vi "ConfigUtilities - Configure Packet Header.vi"(8 "error in (no error)":errorcluster, 9 "Header Elements In":bool[](array[boolean]), 11 "Packet Ref in":T1 format="%.0x") -> (0 "error out":errorcluster, 1 "Header Elements Out":bool[](array[boolean]), 3 "Packet Ref out":T1 format="%.0x")   [LabVIEW 2016, in "UDP-Custom-Device System Explorer.lvlib"]
uses:
  UDP-Custom-Device System Explorer.lvlib
  <vilib>/NI Veristand/Custom Device API/Custom Device Item Ref.ctl
  <vilib>/NI VeriStand/Custom Device API/Custom Device API.lvlib
panel:
  in  "TimeStamp":bool
  out "Data Header":string="Data"
  out "Num Bits Header":string="Num Bits"
  out "Data":string
  out "Num Bits":string
  in  "Cancel":bool
  in  "OK":bool
  in  "Packet Sequence":bool
  in  "Packet ID":bool
  in  "Num of Chans":bool
  # "Select Packet Header Information"
  # "Sample Packet Header"
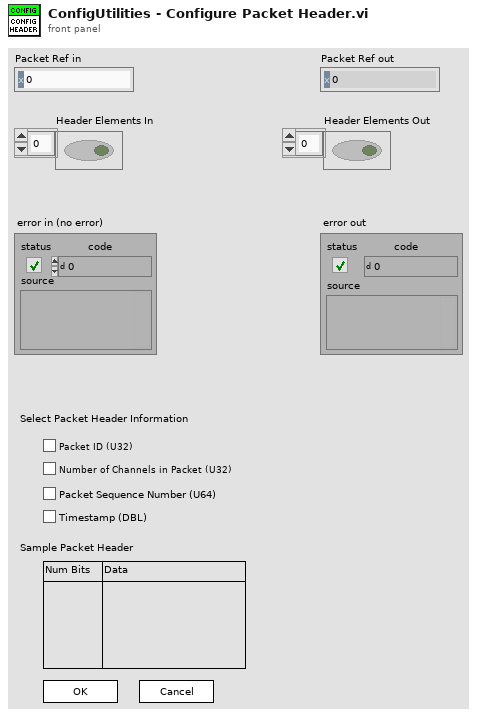
[diagram p1: front panel]
types:
  T1 = typedef "Custom Device API.lvlib/Custom Device Item Ref.ctl" = u64
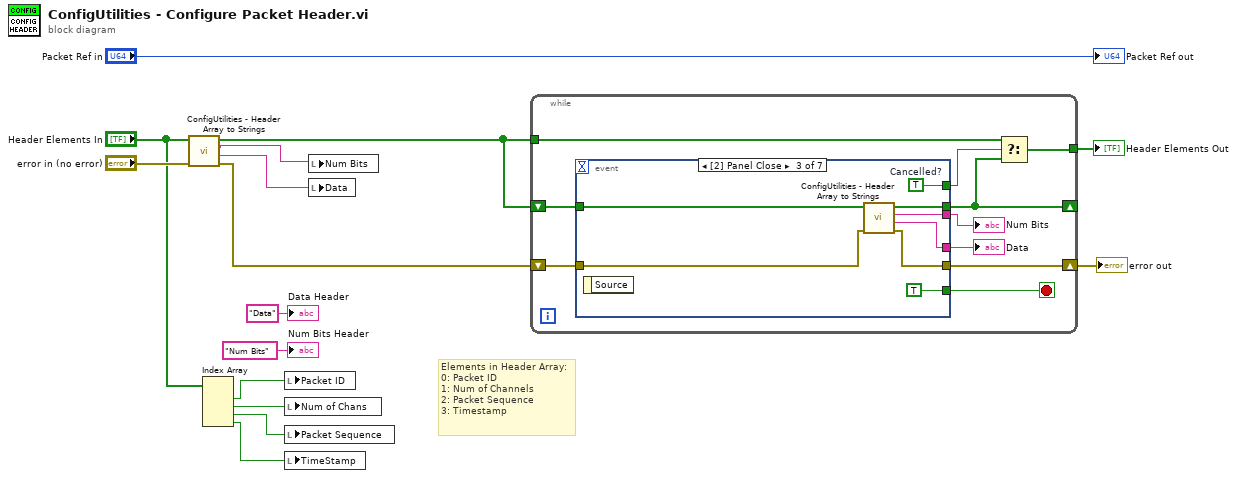
[diagram p0: block diagram]
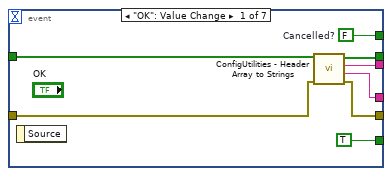
[diagram p2: hidden frame]
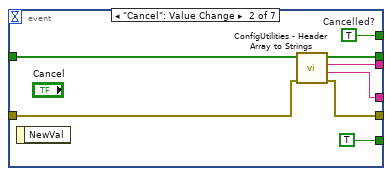
[diagram p3: hidden frame]
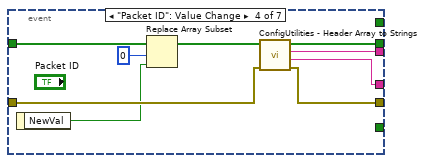
[diagram p4: hidden frame]
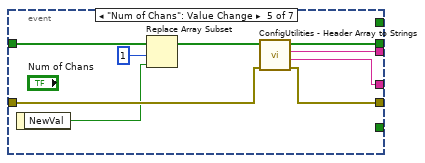
[diagram p5: hidden frame]
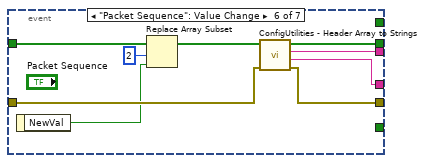
[diagram p6: hidden frame]
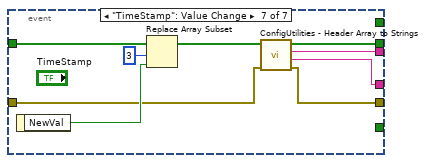
[diagram p7: hidden frame]
diagram:
  # "Elements in Header Array:\n0: Packet ID\n1: Num of Channels\n2: Packet Sequence\n3: Timestamp"
  n1 = call "ConfigUtilities - Header Array to Strings.vi"("error in (no error)"="error in (no error)", "Header Array In"="Header Elements In") -> ("error out"=w1:errorcluster, "Data Name String"=w2:string, "Num Bits String"=w3:string, "Header Array Out"=w4:bool[])  [unwired: 6 in]
  n2 = Index Array(array="Header Elements In") -> (element #1=w9:bool, element #2=w10:bool, element #3=w8:bool, element #4=w7:bool)  [unwired: 4 in]
  n3 = local write "Packet ID"(w9) -> ()
  n4 = local write "Num of Chans"(w10) -> ()
  n5 = local write "Packet Sequence"(w8) -> ()
  n6 = local write "TimeStamp"(w7) -> ()
  n7 = local write "Num Bits"(w3) -> ()
  n8 = local write "Data"(w2) -> ()
  n9 = while {
    tunnel: w4 -> [w23]
    shift-right: [w20] -> _
    shift-left: w4 -> [w25]
    tunnel: [w22] -> w15
    shift-right: [w18] -> w11
    shift-left: w1 -> [w19]
    stop <- w24 stop-if-true
    n10 = event shown="[2] Panel Close" {
      selector: _ -> [_ _ _ _ _ _ _]
      dyn-events: _ -> [_ _ _ _ _ _ _]
      timeout: _ -> [_ _ _ _ _ _ _]
      tunnel: w25 -> [w31 w39 w47 w58 w67 w76 w85]
      tunnel: [w30 w38 w46 w55 w64 w73 w79] -> w20
      tunnel: [w33 w41 w49 _ _ _ _] -> w21
      tunnel: [TRUE TRUE TRUE _ _ _ _] -> w24
      tunnel: w19 -> [w26 w34 w42 w54 w63 w72 w81]
      tunnel: [w28 w36 w44 w53 w62 w71 w80] -> w18
      tunnel: [w29 w37 w45 w52 w61 w70 w78] -> w17
      tunnel: [w27 w35 w43 w51 w60 w69 w77] -> w16
      event "OK": Value Change {
        w33 = FALSE  # Cancelled?
        n11 = event-data() -> ()  [unwired: 1 in, 1 out]
        n12 = call "ConfigUtilities - Header Array to Strings.vi"("error in (no error)"=w26, "Header Array In"=w31) -> ("error out"=w28:errorcluster, "Data Name String"=w27:string, "Num Bits String"=w29:string, "Header Array Out"=w30:bool[])  [unwired: 6 in]
      }
      event "Cancel": Value Change {
        w41 = TRUE  # Cancelled?
        n13 = event-data() -> ()  [unwired: 1 in, 1 out]
        n14 = call "ConfigUtilities - Header Array to Strings.vi"("error in (no error)"=w34, "Header Array In"=w39) -> ("error out"=w36:errorcluster, "Data Name String"=w35:string, "Num Bits String"=w37:string, "Header Array Out"=w38:bool[])  [unwired: 6 in]
      }
      event Panel Close {
        w49 = TRUE  # Cancelled?
        n15 = event-data() -> ()  [unwired: 1 in, 1 out]
        n16 = call "ConfigUtilities - Header Array to Strings.vi"("error in (no error)"=w42, "Header Array In"=w47) -> ("error out"=w44:errorcluster, "Data Name String"=w43:string, "Num Bits String"=w45:string, "Header Array Out"=w46:bool[])  [unwired: 6 in]
      }
      event "Packet ID": Value Change {
        n17 = event-data() -> ("NewVal"=w50:bool)  [unwired: 1 in]
        n18 = Replace Array Subset(array=w58, new element=w50, index=0) -> (w56:bool[])
        n19 = call "ConfigUtilities - Header Array to Strings.vi"("error in (no error)"=w54, "Header Array In"=w56) -> ("error out"=w53:errorcluster, "Data Name String"=w51:string, "Num Bits String"=w52:string, "Header Array Out"=w55:bool[])  [unwired: 6 in]
      }
      event "Num of Chans": Value Change {
        n20 = event-data() -> ("NewVal"=w59:bool)  [unwired: 1 in]
        n21 = Replace Array Subset(array=w67, new element=w59, index=1) -> (w65:bool[])
        n22 = call "ConfigUtilities - Header Array to Strings.vi"("error in (no error)"=w63, "Header Array In"=w65) -> ("error out"=w62:errorcluster, "Data Name String"=w60:string, "Num Bits String"=w61:string, "Header Array Out"=w64:bool[])  [unwired: 6 in]
      }
      event "Packet Sequence": Value Change {
        n23 = event-data() -> ("NewVal"=w68:bool)  [unwired: 1 in]
        n24 = Replace Array Subset(array=w76, new element=w68, index=2) -> (w74:bool[])
        n25 = call "ConfigUtilities - Header Array to Strings.vi"("error in (no error)"=w72, "Header Array In"=w74) -> ("error out"=w71:errorcluster, "Data Name String"=w69:string, "Num Bits String"=w70:string, "Header Array Out"=w73:bool[])  [unwired: 6 in]
      }
      event "TimeStamp": Value Change {
        n26 = event-data() -> ("NewVal"=w83:bool)  [unwired: 1 in]
        n27 = Replace Array Subset(array=w85, new element=w83, index=3) -> (w82:bool[])
        n28 = call "ConfigUtilities - Header Array to Strings.vi"("error in (no error)"=w81, "Header Array In"=w82) -> ("error out"=w80:errorcluster, "Data Name String"=w77:string, "Num Bits String"=w78:string, "Header Array Out"=w79:bool[])  [unwired: 6 in]
      }
    }
    "Num Bits" <- w17
    "Data" <- w16
    n29 = Select(t=w23, s=w21, f=w20) -> (s? t:f=w22:bool[])
  }
  "error out" <- w11
  "Header Elements Out" <- w15
  "Packet Ref out" <- "Packet Ref in"
  "Num Bits Header" <- "Num Bits" ("Num Bits Header")
  "Data Header" <- "Data" ("Data Header")
